vi "Configure Sequencer List Filling Digital Gain.vi"(7 "Increment (0.0)":dbl format="%^.3e", 8 "error in (no error)":errorcluster, 9 "Start Value (0.0)":dbl format="%^.3e", 10 "Instance (1)":i32=1, 11 "VISA resource name":refnum<visa-resource-name>) -> (0 "error out":errorcluster, 3 "VISA resource name out":refnum<visa-resource-name>)   [LabVIEW 2020, in "Rohde&Schwarz CMXP GPRF.lvlib"]
doc: "Configures values for filling the sequencer list with digital gain values.\n\nAttributes:\nRSCMXPGPRF_ATTR_SEQUENCER_LIST_FILLING_DIGITAL_GAIN_START_VALUE\nRSCMXPGPRF_ATTR_SEQUENCER_LIST_FILLING_DIGITAL_GAIN_INCREMENT\n\nRemote-control commands:\nSOURce:GPRF:GEN<i>:SEQuencer:LIST:FILL:DGAin:SVALue\nSOURce:GPRF:GEN<i>:SEQuencer:LIST:FILL:DGAin:INCRement"
uses:
  <instrlib>/Rohde&Schwarz CMXP GPRF/Rohde&Schwarz CMXP GPRF.lvlib
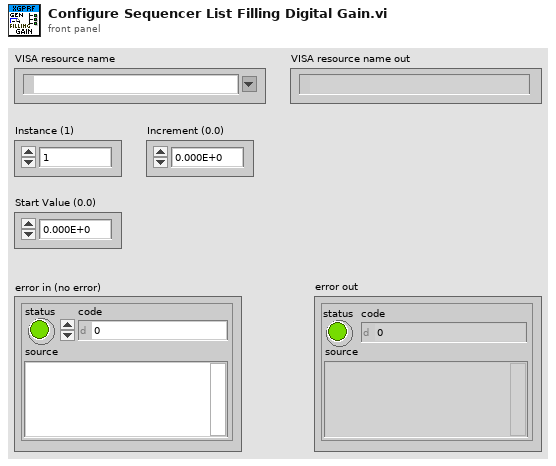
[diagram p1: front panel]
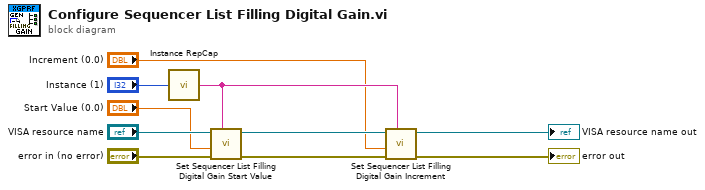
[diagram p0: block diagram]
diagram:
  n1 = call <instrlib>:"Instance RepCap.vi"("Instance in"="Instance (1)") -> ("Instance out"=w3:string)
  n2 = call "Set Sequencer List Filling Digital Gain Start Value"("Repeated Capabilities"=w3, "error in (no error)"="error in (no error)", "Sequencer List Filling Digital Gain Start Value (0.0)"="Start Value (0.0)", "instrument handle"="VISA resource name") -> ("error out"=w5:errorcluster, "instrument handle out"=w6:refnum<visa-resource-name>)  [unwired: 6 in]
  n3 = call "Set Sequencer List Filling Digital Gain Increment"("Repeated Capabilities"=w3, "error in (no error)"=w5, "Sequencer List Filling Digital Gain Increment (0.0)"="Increment (0.0)", "instrument handle"=w6) -> ("error out"=→"error out":errorcluster, "instrument handle out"=→"VISA resource name out":refnum<visa-resource-name>)  [unwired: 6 in]
